vi "Fit Transform.vi"(7 "Type X":T1(ring), 8 "error in (no error)":errorcluster caption="entrée d'erreur (pas d'erreur)", 9 "y":string[][](array[string]), 10 "X":string[][](array[string]), 11 "FunctionTransformer.lvclass":refnum<class "FunctionTransformer.lvclass">) -> (0 "error in (no error)":errorcluster caption="entrée d'erreur (pas d'erreur)", 2 "Data":T2, 3 "FunctionTransformer.lvclass":refnum<class "FunctionTransformer.lvclass">)   [LabVIEW 2020, in "FunctionTransformer.lvclass"]
doc: "Fit to data, then transform it.\n\nFits transformer to X and y with optional parameters fit_params and returns a transformed version of X.\n\nReturns : \n\n- X_new : ndarray array of shape (n_samples, n_features_new)\nTransformed array."
uses:
  FunctionTransformer.lvclass
  FunctionTransformer.lvclass/FunctionTransformer.ctl
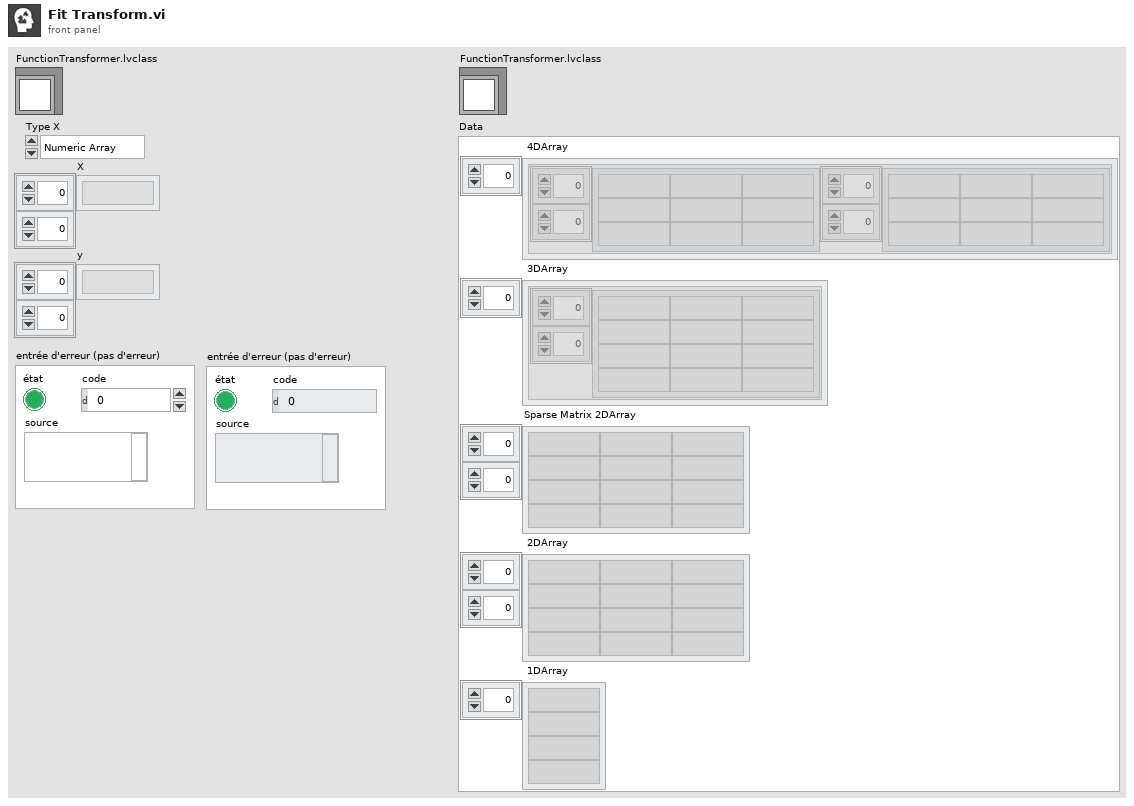
[diagram p1: front panel]
types:
  T1 = enum16{"Numeric Array", "String Array", "Sparse"}
  T2 = cluster{" 4DArray":cluster{"1":string[][], "2":string[][]}[], " 3DArray":cluster{"Tableau":string[][]}[], "Sparse Matrix 2DArray":string[][], " 2DArray":string[][], " 1DArray":string[]}
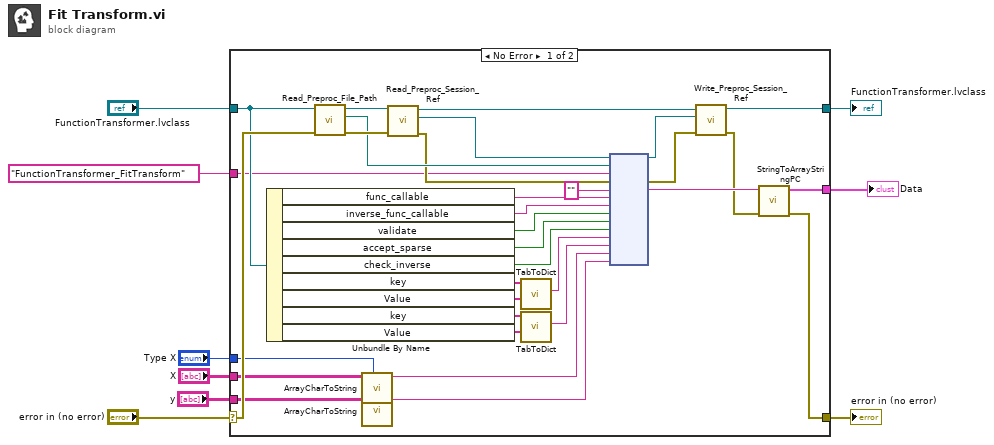
[diagram p0: block diagram]
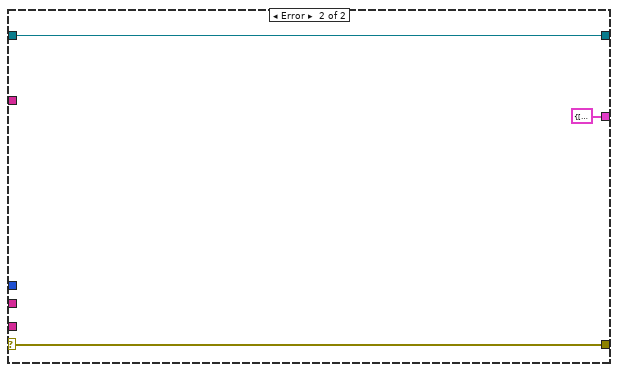
[diagram p2: hidden frame]
diagram:
  n1 = case shown="No Error" "error in (no error)" {
    selector: "error in (no error)" -> [w33 w45]
    tunnel: [w21 w45] -> w8
    tunnel: [w22 w44] -> w6
    tunnel: "FunctionTransformer.lvclass" -> [w32 w44]
    tunnel: "FunctionTransformer_FitTransform" ("Fonction") -> [w26 _]
    tunnel: [w24 T2 {" 4DArray"=[], " 3DArray"=[], "Sparse Matrix 2DArray"=[], " 2DArray"=[], " 1DArray"=[]} ("Data")] -> w4
    tunnel: "X" -> [w20 _]
    tunnel: "y" -> [w18 _]
    tunnel: "Type X" -> [w10 _]
    frame No Error {
      n2 = Unbundle By Name(w32) -> ("func_callable"=w31:string, "inverse_func_callable"=w30:string, "validate"=w29:bool, "accept_sparse"=w28:bool, "check_inverse"=w27:bool, "key"=w16:string[], "Value"=w15:string[], "key"=w14:string[], "Value"=w13:string[])
      n3 = call-dynamic "Read_Preproc_File_Path.vi"("error in (no error)"=w33, "Python in"=w32) -> ("error out"=w41:errorcluster, "File_Path"=w38:path, "Python out"=w42:refnum<class "FunctionTransformer.lvclass">)  [unwired: 7 in]
      n4 = call "ArrayCharToString.vi"("Type"=w10, "TAB"=w20) -> ("Instruction"=w19:string)  [unwired: 9 in]
      n5 = call "ArrayCharToString.vi"("TAB"=w18) -> ("Instruction"=w17:string)  [unwired: 10 in]
      n6 = call-dynamic "Read_Preproc_Session_Ref.vi"("error in (no error)"=w41, "Python in"=w42) -> ("error out"=w37:errorcluster, "Session_ref"=w39:refnum<k35>, "Python out"=w40:refnum<class "FunctionTransformer.lvclass">)  [unwired: 7 in]
      n7 = call "TabToDict.vi"("String Value"=w15, "String key"=w16) -> ("Dict with string value"=w11:string)  [unwired: 8 in, 1 out]
      n8 = call "TabToDict.vi"("String Value"=w13, "String key"=w14) -> ("Dict with string value"=w12:string)  [unwired: 8 in, 1 out]
      n9 = node(w39, w38, w26, w37, "", w31, w30, w29, w28, w27, w11, w12, w19, w17) -> (w35:refnum<k35>, w36:errorcluster, w25:string)  [unwired: 9 in, 2 out]
      n10 = call-dynamic "Write_Preproc_Session_Ref.vi"("error in (no error)"=w36, "Session_ref"=w35, "Python in"=w40) -> ("error out"=w23:errorcluster, "Python out"=w22:refnum<class "FunctionTransformer.lvclass">)  [unwired: 7 in]
      n11 = call "StringToArrayStringPC.vi"("sortie d'erreur"=w23, "Return value"=w25) -> ("sortie d'erreur"=w21:errorcluster, "Data"=w24:T2)  [unwired: 8 in]
    }
    frame Error {
    }
  }
  "error in (no error)" <- w8
  "FunctionTransformer.lvclass" <- w6
  "Data" <- w4
